vi "PSAE_VCH_Get VCHs Enabled.vi"(8 "Error In (no error)":errorcluster, 11 "VCH":T1) -> (0 "Error Out":errorcluster, 3 "VCH":T1)   [LabVIEW 2016]
uses:
  VCH/Private/Ctrls/PSVCH_VCH Info.ctl
panel:
  # "Data In"
  # "Data Out"
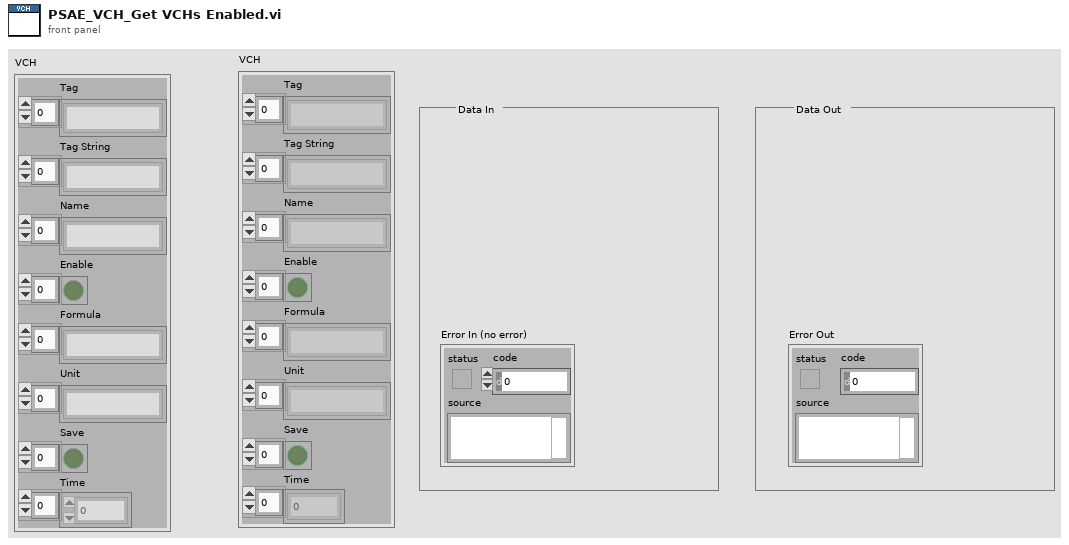
[diagram p1: front panel]
types:
  T1 = typedef "PSVCH_VCH Info.ctl" = cluster{"Tag":string[], "Tag String":string[], "Name":string[], "Enable":bool[], "Formula":string[], "Unit":string[], "Save":bool[], "Time":i64[]}
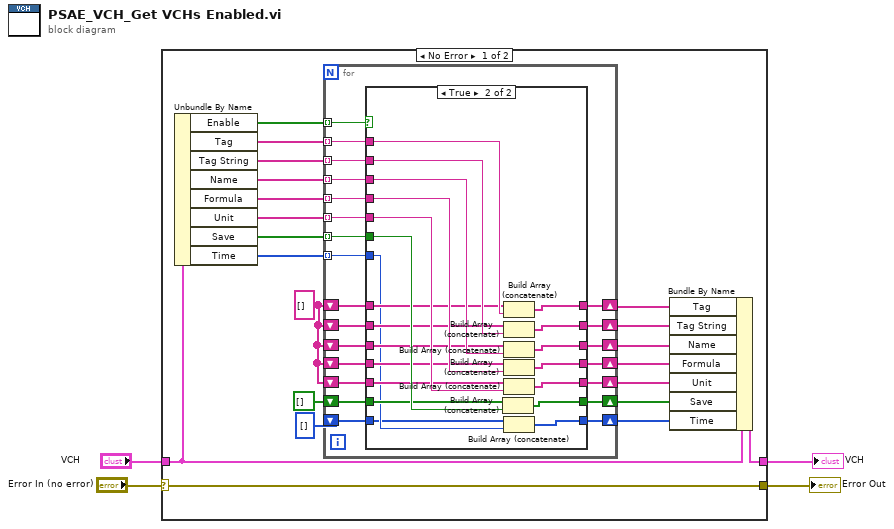
[diagram p0: block diagram]
diagram:
  n1 = case shown="No Error" "Error In (no error)" {
    selector: "Error In (no error)" -> [w25 w77]
    tunnel: [w25 w77] -> w3
    tunnel: "VCH" -> [w17 w76]
    tunnel: [w16 w76] -> w1
    frame No Error {
      w8 = string[] []
      n2 = Unbundle By Name(w17) -> ("Enable"=w18:bool[], "Tag"=w19:string[], "Tag String"=w20:string[], "Name"=w21:string[], "Formula"=w22:string[], "Unit"=w23:string[], "Save"=w24:bool[], "Time"=w7:i64[])
      n3 = for {
        tunnel: w18 -> [w47] mode=indexing
        tunnel: w19 -> [w46] mode=indexing
        tunnel: w20 -> [w45] mode=indexing
        tunnel: w21 -> [w44] mode=indexing
        tunnel: w22 -> [w43] mode=indexing
        tunnel: w23 -> [w42] mode=indexing
        tunnel: w24 -> [w41] mode=indexing
        shift-right: [w40] -> w15
        shift-left: w8 -> [w39]
        shift-right: [w38] -> w14
        shift-left: w8 -> [w37]
        shift-right: [w36] -> w13
        shift-left: w8 -> [w35]
        shift-right: [w34] -> w12
        shift-left: w8 -> [w33]
        shift-right: [w32] -> w11
        shift-left: w8 -> [w31]
        shift-right: [w30] -> w10
        shift-left: bool[] [] -> [w29]
        shift-right: [w28] -> w6
        shift-left: i64[] [] -> [w26]
        tunnel: w7 -> [w27] mode=indexing
        n4 = case shown="True" w47 {
          tunnel: w46 -> [_ w75]
          tunnel: w45 -> [_ w74]
          tunnel: w44 -> [_ w73]
          tunnel: w43 -> [_ w72]
          tunnel: w42 -> [_ w71]
          tunnel: w41 -> [_ w70]
          tunnel: [w54 w69] -> w40
          tunnel: w39 -> [w54 w68]
          tunnel: [w53 w67] -> w38
          tunnel: w37 -> [w53 w66]
          tunnel: [w52 w65] -> w36
          tunnel: w35 -> [w52 w64]
          tunnel: [w51 w63] -> w34
          tunnel: w33 -> [w51 w62]
          tunnel: [w50 w61] -> w32
          tunnel: w31 -> [w50 w60]
          tunnel: [w49 w59] -> w30
          tunnel: w29 -> [w49 w58]
          tunnel: [w48 w57] -> w28
          tunnel: w27 -> [_ w56]
          tunnel: w26 -> [w48 w55]
          frame False {
          }
          frame True {
            n5 = Build Array (concatenate)(w58, w70) -> (w59:bool[])
            n6 = Build Array (concatenate)(w68, w75) -> (w69:string[])
            n7 = Build Array (concatenate)(w66, w74) -> (w67:string[])
            n8 = Build Array (concatenate)(w64, w73) -> (w65:string[])
            n9 = Build Array (concatenate)(w62, w72) -> (w63:string[])
            n10 = Build Array (concatenate)(w60, w71) -> (w61:string[])
            n11 = Build Array (concatenate)(w55, w56) -> (w57:i64[])
          }
        }
      }
      n12 = Bundle By Name(cluster=w17, "Tag"=w15, "Tag String"=w14, "Name"=w13, "Formula"=w12, "Unit"=w11, "Save"=w10, "Time"=w6) -> (w16:T1)
    }
    frame Error {
    }
  }
  "VCH" <- w1
  "Error Out" <- w3
